vi "iRobot UART Read.vi"(8 "error in":errorcluster, 11 "UART port in":T1) -> (0 "error out":errorcluster, 1 "data":u8[](array[numeric]), 3 "UART port out":T1)   [LabVIEW 2010]
doc: "Read all available data from the UART receive buffer."
uses:
  UART Port Type.ctl
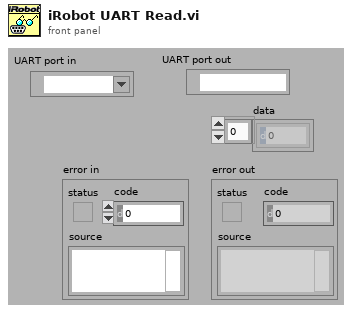
[diagram p1: front panel]
types:
  T1 = typedef "UART Port Type.ctl" = refnum<visa-resource-name>
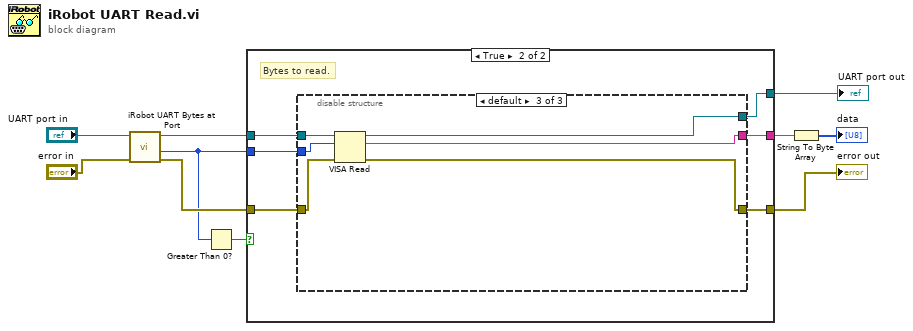
[diagram p0: block diagram]
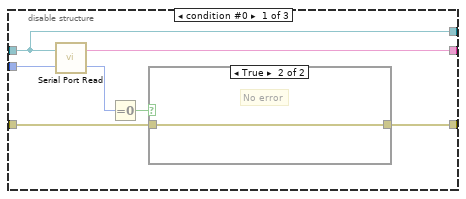
[diagram p3: hidden frame]
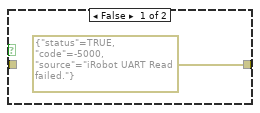
[diagram p4: hidden frame]
diagram:
  n1 = call "iRobot UART Bytes at Port.vi"("error in"="error in", "UART port in"="UART port in") -> ("error out"=w5:errorcluster, "bytes at port"=w4:u32, "UART port out"=w6:T1)  [unwired: 1 in, 6 out]
  n2 = Greater Than 0?(x=w4) -> (x > 0?=w3:bool)
  n3 = case shown="True" w3 {
    tunnel: w6 -> [w11 w18]
    tunnel: w4 -> [_ w17]
    tunnel: [_ w16] -> w2
    tunnel: w5 -> [w12 w15]
    tunnel: [w12 w14] -> w9
    tunnel: [w11 w13] -> w1
    frame False {
      # "No bytes at port."
    }
    frame True {
      # "Bytes to read."
      n4 = disable-structure shown="default" {
        disable-tunnel: w18 -> [w19 _ w33]
        disable-tunnel: w17 -> [w25 _ w32]
        disable-tunnel: [w24 _ w29] -> w16
        disable-tunnel: w15 -> [w21 _ w31]
        disable-tunnel: [w20 _ w28] -> w14
        disable-tunnel: [w19 _ w30] -> w13
        frame condition #0 {
          n5 = call <vilib>:"Serial Port Read.vi"("requested byte count"=w25, "port number"=w19) -> ("error code"=w22:i32, "string read"=w24:string)
          n6 = Equal To 0?(x=w22) -> (x = 0?=w23:bool)
          n7 = case shown="True" w23 {
            tunnel: [errorcluster {"status"=TRUE, "code"=-5000, "source"="iRobot UART Read failed."} ("error out") w27] -> w20
            tunnel: w21 -> [_ w27]
            frame False {
            }
            frame True {
              # "No error"
            }
          }
        }
        frame condition #1 {
          # "To be deployed..."
        }
        frame condition #2 (active) {
          n8 = VISA Read(VISA resource name=w33, byte count=w32, error in (no error)=w31) -> (VISA resource name out=w30:T1, read buffer=w29:string, error out=w28:errorcluster)  [unwired: 1 out]
        }
      }
    }
  }
  "UART port out" <- w1
  "error out" <- w9
  n9 = String To Byte Array(string=w2) -> (unsigned byte array=→"data":u8[])
